vi "Find Routing and Faulting Custom Device.vi"(8 "error in (no error)":errorcluster, 11 "Target in":refnum<k24>) -> (0 "error out":errorcluster, 2 "Routing and Faulting Custom Device Ref":T1 format="%.0x", 3 "Target out":refnum<k24>)   [LabVIEW 2017, in "Routing and Faulting Scripting.lvlib"]
uses:
  Routing and Faulting Scripting.lvlib
  NationalInstruments.VeriStand.SystemDefinitionAPI
  <vilib>/NI Veristand/Custom Device API/Custom Device Item Ref.ctl
  Shared/Constants.vi
  Shared/Routing and Faulting Shared.lvlib
  <vilib>/NI VeriStand/Custom Device API/Custom Device API.lvlib
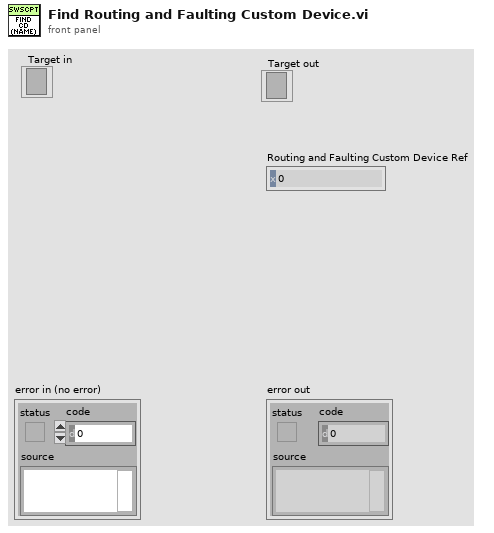
[diagram p1: front panel]
types:
  T1 = typedef "Custom Device API.lvlib/Custom Device Item Ref.ctl" = u64
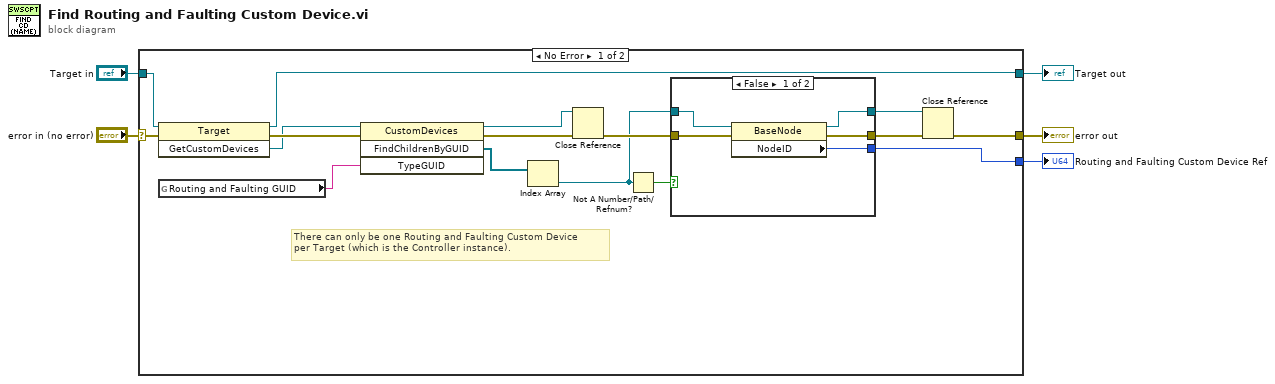
[diagram p0: block diagram]
diagram:
  n1 = case shown="No Error" "error in (no error)" {
    selector: "error in (no error)" -> [w21 w30]
    tunnel: [w10 w30] -> w5
    tunnel: "Target in" -> [w20 w29]
    tunnel: [w14 w29] -> w2
    tunnel: [w12 _] -> w1
    frame No Error {
      # "There can only be one Routing and Faulting Custom Device\nper Target (which is the Controller instance)."
      n2 = invoke class="Target" method="GetCustomDevices"(reference=w20, error in=w21) -> (reference out=w14:refnum<k24>, error out=w19:errorcluster, "GetCustomDevices"=w18:refnum<k24>)  [unwired: 1 in]
      n3 = global read "Constants.vi" "Routing and Faulting GUID"() -> (w8:string)
      n4 = invoke class="CustomDevices" method="FindChildrenByGUID"(reference=w18, error in=w19, "TypeGUID"=w8) -> (reference out=w17:refnum<k24>, error out=w16:errorcluster, "FindChildrenByGUID"=w7:refnum<k24>[])  [unwired: 1 in, 1 out]
      n5 = Index Array(array=w7) -> (element=w6:refnum<k24>)  [unwired: 1 in]
      n6 = Close Reference(reference=w17, error in (no error)=w16) -> (error out=w15:errorcluster)
      n7 = Not A Number/Path/Refnum?(number/path/refnum=w6) -> (NaN/Path/Refnum?=w13:bool)
      n8 = case shown="False" w13 {
        tunnel: [w22 w28] -> w9
        tunnel: w15 -> [w24 w28]
        tunnel: w6 -> [w26 w27]
        tunnel: [w25 _] -> w12
        tunnel: [w23 w27] -> w11
        frame False {
          n9 = property class="BaseNode"(reference=w26, error in=w24) -> (reference out=w23:refnum<k24>, error out=w22:errorcluster, "NodeID"=w25:u64)
        }
        frame True {
        }
      }
      n10 = Close Reference(reference=w11, error in (no error)=w9) -> (error out=w10:errorcluster)
    }
    frame Error {
    }
  }
  "Target out" <- w2
  "error out" <- w5
  "Routing and Faulting Custom Device Ref" <- w1
